vi "Code Conversion Paths.vi"(11 "error in":errorcluster) -> (2 "folders to ignore":path, 3 "deafult value setter vi":path, 4 "is project directory":path, 6 "io controls":path, 8 "get resource vi":path, 10 "error log path":path, 13 "deserializer":path, 14 "serializer":path, 15 "error out":errorcluster)   [LabVIEW 2021, in "Path Functions.lvlib"]
uses:
  Path Functions.lvlib
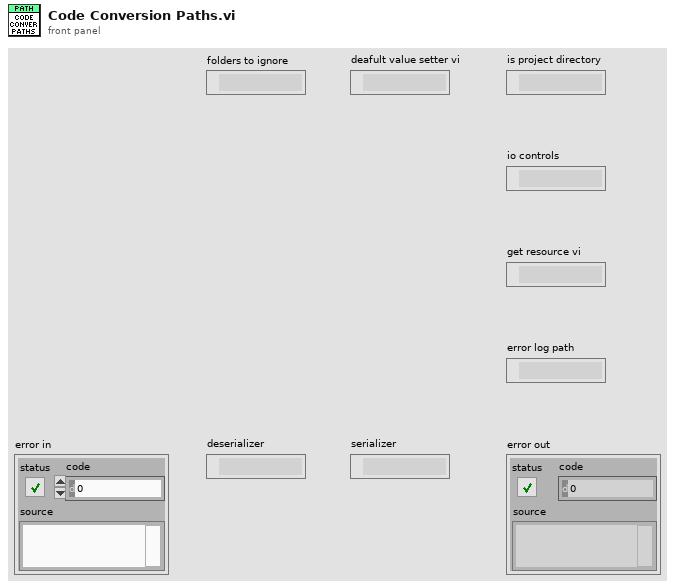
[diagram p1: front panel]
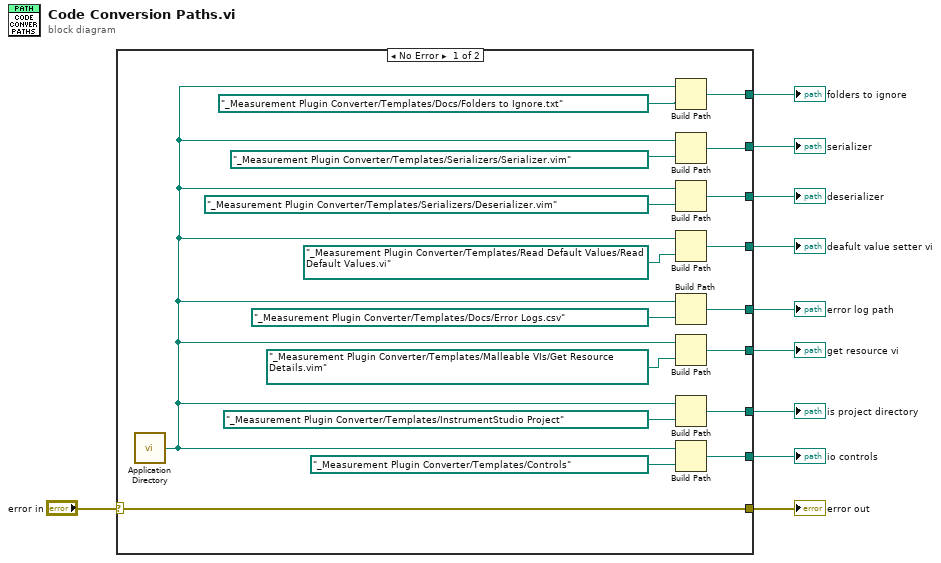
[diagram p0: block diagram]
diagram:
  n1 = case shown="No Error" "error in" {
    selector: "error in" -> [w23 w29]
    tunnel: [w28 _] -> w10
    tunnel: [w27 _] -> w9
    tunnel: [w26 _] -> w8
    tunnel: [w24 _] -> w7
    tunnel: [w18 _] -> w6
    tunnel: [w23 w29] -> w5
    tunnel: [w20 _] -> w4
    tunnel: [w19 _] -> w3
    tunnel: [w15 _] -> w2
    frame No Error {
      n2 = call <vilib>:"Application Directory.vi"() -> ("Application Directory"=w17:path)
      n3 = Build Path(base path=w17, name or relative path=path "_Measurement Plugin Converter/Templates/Docs/Folders to Ignore.txt") -> (appended path=w15:path)
      n4 = Build Path(base path=w17, name or relative path=path "_Measurement Plugin Converter/Templates/Serializers/Serializer.vim") -> (appended path=w18:path)
      n5 = Build Path(base path=w17, name or relative path=path "_Measurement Plugin Converter/Templates/Serializers/Deserializer.vim") -> (appended path=w20:path)
      n6 = Build Path(base path=w17, name or relative path=path "_Measurement Plugin Converter/Templates/Read Default Values/Read Default Values.vi") -> (appended path=w19:path)
      n7 = Build Path(base path=w17, name or relative path=path "_Measurement Plugin Converter/Templates/Docs/Error Logs.csv") -> (appended path=w24:path)
      n8 = Build Path(base path=w17, name or relative path=path "_Measurement Plugin Converter/Templates/Malleable VIs/Get Resource Details.vim") -> (appended path=w26:path)
      n9 = Build Path(base path=w17, name or relative path=path "_Measurement Plugin Converter/Templates/InstrumentStudio Project") -> (appended path=w28:path)
      n10 = Build Path(base path=w17, name or relative path=path "_Measurement Plugin Converter/Templates/Controls") -> (appended path=w27:path)
    }
    frame Error {
    }
  }
  "error out" <- w5
  "is project directory" <- w10
  "io controls" <- w9
  "get resource vi" <- w8
  "error log path" <- w7
  "deserializer" <- w4
  "serializer" <- w6
  "deafult value setter vi" <- w3
  "folders to ignore" <- w2
